vi "CalcGaitTiming.vi"() -> ()   [LabVIEW 2015]
uses:
  Classes/CAlex_Classes/CAlexData2/CAlexData2.lvclass
  <vilib>/Utility/file.llb/Write To Spreadsheet File (string).vi
panel:
  in  "Multicolumn Listbox":i32(listbox)
  in  "File Name":string
  out "Stance/Swing":dbl format="%0.2f"
  out "SwingTime":dbl format="%0.2f"
  out "GaitTime":dbl format="%0.2f"
  out "Total":i32
  out "Current":i32
  in  "pattern":string
  in  "Path":path
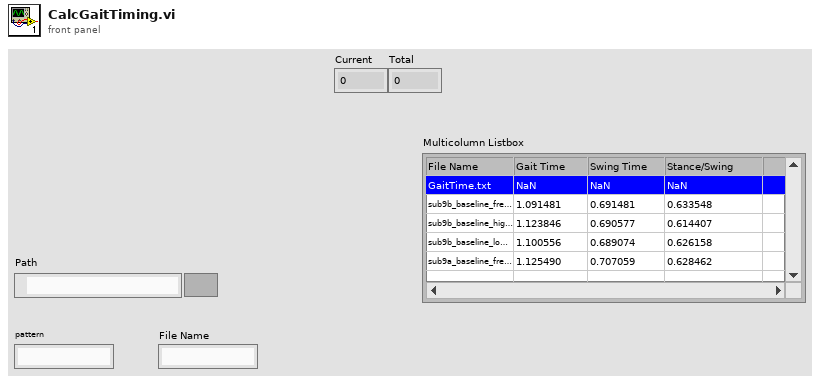
[diagram p1: front panel]
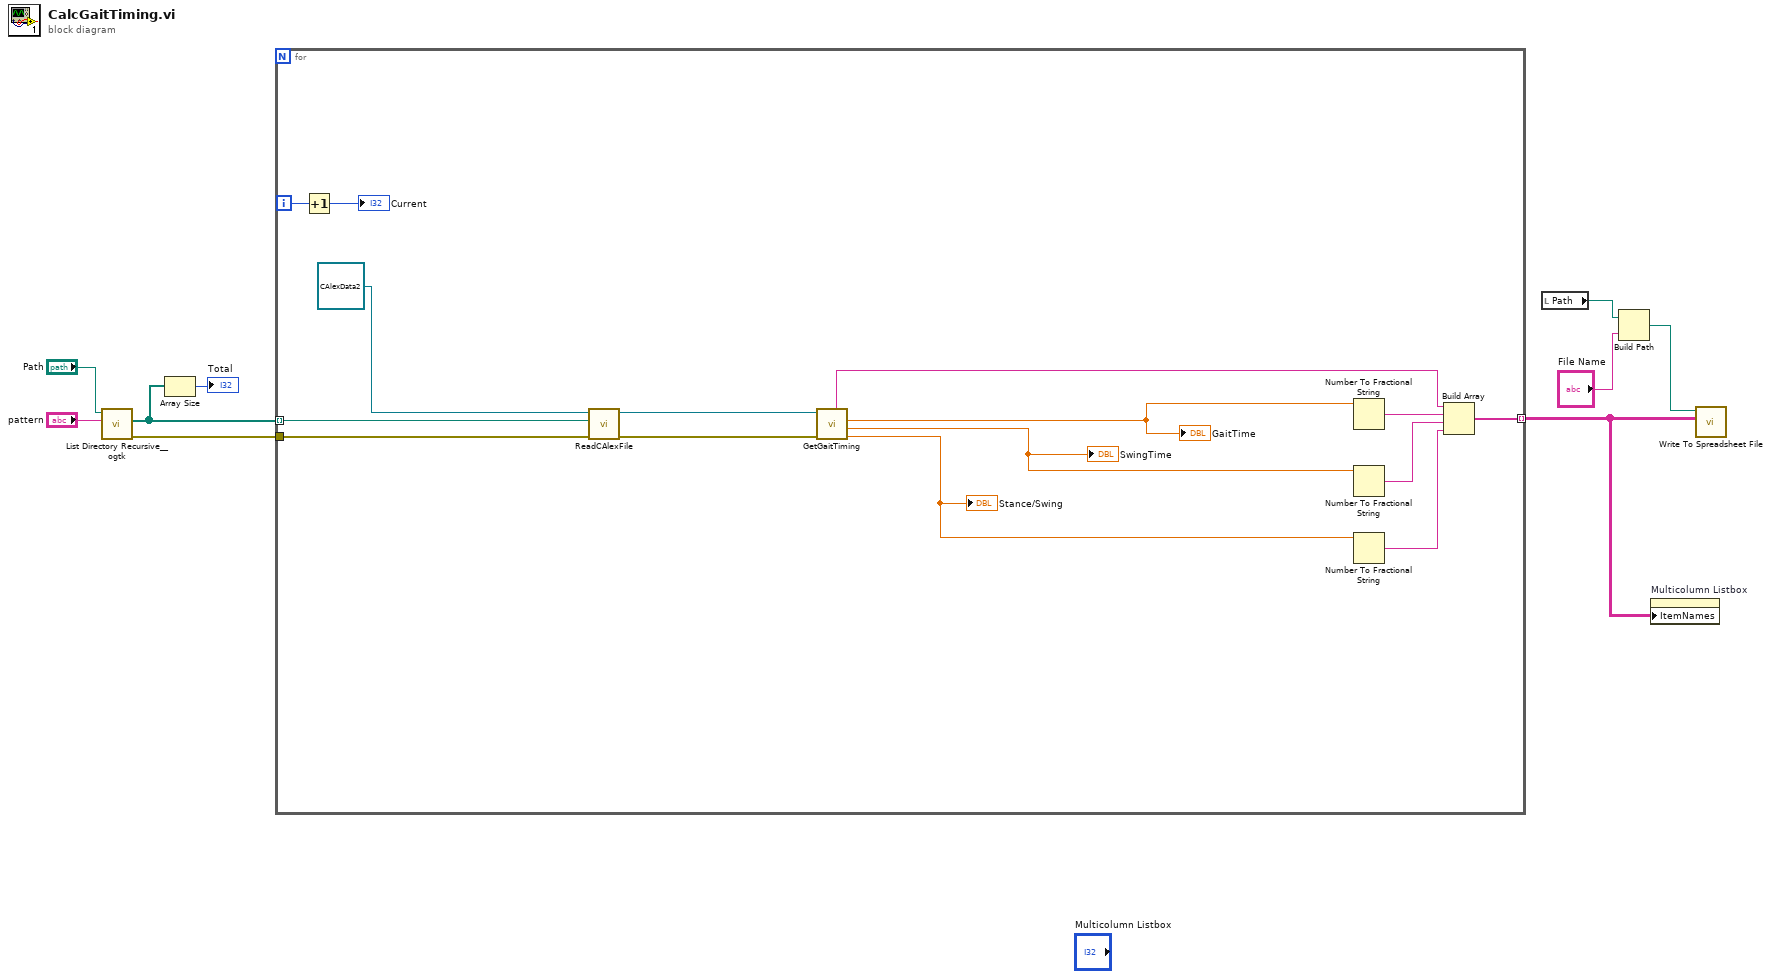
[diagram p0: block diagram]
diagram:
  n1 = call <userlib>:"List Directory Recursive__ogtk.vi"("pattern"="pattern", "Path"="Path") -> ("error out"=w7:errorcluster, "file paths"=w6:path[])  [unwired: 6 in, 2 out]
  n2 = Array Size(array=w6) -> (size(s)=→"Total":i32)
  n3 = for {
    tunnel: w6 -> [w10] mode=indexing
    tunnel: w7 -> [w13]
    tunnel: [w19] -> w1 mode=indexing
    i -> [w24]
    n4 = Increment(x=w24) -> (x+1=→"Current":i32)
    n5 = call "ReadCAlexFile.vi"("error in (no error)"=w13, "ExpData File Path"=w10, "CAlexData2"=refnum<class "CAlexData2.lvclass"> refnum) -> ("error out"=w11:errorcluster, "CAlexData 2"=w12:refnum<class "CAlexData2.lvclass">)  [unwired: 7 in]
    n6 = call "GetGaitTiming.vi"("error in (no error)"=w11, "CAlexData2 in"=w12) -> ("Stance/Swing"=w16:dbl, "SwingTime"=w17:dbl, "GaitTime"=w18:dbl, "FileName"=w15:string)  [unwired: 5 in, 1 out]
    "GaitTime" <- w18
    "SwingTime" <- w17
    "Stance/Swing" <- w16
    n7 = Number To Fractional String(number=w18) -> (F-format string=w22:string)  [unwired: 3 in]
    n8 = Number To Fractional String(number=w17) -> (F-format string=w21:string)  [unwired: 3 in]
    n9 = Number To Fractional String(number=w16) -> (F-format string=w20:string)  [unwired: 3 in]
    n10 = Build Array(w15, w22, w21, w20) -> (w19:string[])
  }
  n11 = local read "Path"() -> (w4:path)
  n12 = Build Path(base path=w4, name or relative path="File Name") -> (appended path=w2:path)
  n13 = property on="Multicolumn Listbox" class="MCListbox (strict)"("ItemNames"=w1) -> ()  [unwired: 2 in, 2 out]
  n14 = call-poly <vilib>:"Write To Spreadsheet File.vi"("2D data"=w1, "file path (dialog if empty)"=w2) -> ()  [unwired: 6 in, 1 out]
